vi "Sweep Control.vi"(1 "Stop":bool, 4 "Experiment Description":string="IV measurements at 0T\n- Sweep priority 0: +x gate from -10V to 10V in steps of 500mV (-x 10 to -10)\n- priority 1:+y gate from -10V to 10V in steps of 500mV (-y 10 to -10)\n- 1 IV curves at each Vsg\n- KH channel 17,18,19,20: leads 3,8,15,21\n- 5 s wait\n\nVbg = lead 26: 0V\nT: 20mK\nB=0T\n\nhash device\n\nKH channel 10,13: leads 16,27 , current mode, 5k resistor, 1000x gain\nlead 16: 3mV ac+ 1mV dc bias, 1 Hz\nKH channel 11,12: V1+/-: 17/20, 100x gain\nKH channel 5: dV: 17-20, 100x gain\n\nstripe device\n\nKH channel 7,8: leads 11,12 , current mode, 5k resistor, 1000x gain\nlead 12: 3.5mV ac+ 0mV dc bias, 1 Hz\nKH channel 6,9: V1+/-: 9,13, 100x gain\nKH channel 16: dV: 11-12, 100x gain", 5 "Experiment subVI":T6, 7 "Experiment Folder (## - Description)":string="35-2D_0T_IV_hash_stripe", 8 "error in (no error)":errorcluster, 9 "Post action (indexing priority)":T7=[enum."Do Nothing", enum."Do Nothing", enum."Do Nothing", enum."Do Nothing"], 10 "Scan parameters":T8=[{"Start"=0.0, "End"=0.0, "Step"=0.0, "Rate"=0.0, "Waveform type"=enum."linear", "wait (ms or K)"=0.0, "Address"="Dev2/ao0", "channel"=17}, {"Start"=0.0, "End"=0.0, "Step"=0.0, "Rate"=0.0, "Waveform type"=enum."linear", "wait (ms or K)"=0.0, "Address"="Dev2/ao0", "channel"=18}, {"Start"=0.0, "End"=0.0, "Step"=0.0, "Rate"=0.0, "Waveform type"=enum."linear", "wait (ms or K)"=0.0, "Address"="Dev2/ao0", "channel"=19}, {"Start"=0.0, "End"=0.0, "Step"=0.0, "Rate"=0.0, "Waveform type"=enum."linear", "wait (ms or K)"=0.0, "Address"="Dev2/ao0", "channel"=20}] {"Rate" format="%.2f"; "Step" format="%#_6p"; "End" format="%#_6p"; "Start" format="%#_6p"}, 11 "Scan control":T10=[{"Priority"=enum."Priority 0", "Scan name"=enum."Lockin Bias"}, {"Priority"=enum."Priority 1", "Scan name"=enum."Lockin Bias"}, {"Priority"=enum."Priority 0", "Scan name"=enum."Lockin Bias"}, {"Priority"=enum."Priority 1", "Scan name"=enum."Lockin Bias"}]) -> (0 "error out":errorcluster)   [LabVIEW 2019, in "Sweep Control.lvclass"]
doc: "- Priority 0 is the fastest loop\n- You can put multiple scan names in one priority.\n- OFF has to be the last priority\n- Choose an Experiment (Lockin_Sweep, IV, etc) to run at each Scan Setting\n- Open the Exeriment subVIs to choose settings"
uses:
  Sweep Control.lvclass
  Typedefs/Enum - Priority.ctl
  Typedefs/Enum - Action.ctl
  Typedefs/Cluster - ScanControl.ctl
  Typedefs/ScanControl.ctl
  Typedefs/Cluster - ScanParamters.ctl
  Typedefs/ScanParamters.ctl
  Typedefs/Enum - Experiments.ctl
  Typedefs/Sweep Control JSON--Cluster.ctl
  <userlib>/LevyLab/Transport/Control Experiment/Control Experiment.lvclass
  <userlib>/LevyLab/Transport/Transport/Transport.lvclass
  61c560dc-d997-4a5c-883d-5fdd7af828d2.vi
  Typedefs/PostAction.ctl
  Typedefs/Enum - PostAction.ctl
  Typedefs/Cluster - Sweep Control.ctl
  <userlib>/LevyLab/Transport/Transport/Typedefs/Lockin_Sweep JSON--Cluster.ctl
panel:
  in  "Lockin_Sweep Configuration":T1[](array[typedef]) {"sweepTables"."Table" format="%#_3p"; "sweepTables"."Ch" min=1 max=16; "sweepChannels"."Table" format="%#_1f"; "sweepChannels"."Channel" min=1 max=128; "sweepChannels"."Start" format="%#_6p"; "sweepChannels"."End" format="%#_6p"}
  out "Repeat #":i32
  in  "Repeat Experiment":i32=1 caption="Repeat Experiment (at each parameter)" min=1
  in  "Scan parameters 2":T2[](array[typedef]) {"Rate" format="%.2f"; "Step" format="%#_6p"; "End" format="%#_6p"; "Start" format="%#_6p"}
  # "1. Scan Parameters. Choose parameters at which each experiment will take place."
  # "2. Experiment"
  # "3. If your chosen experiment is \"Lockin Sweep\", then the following sequence of sweeps will be executed at each scan parameter. (Ex. 1. Set B. 2. Set Set Vsg. 3. Lockin Sweep 1. 4. Lockin Sweep 2. Etc."
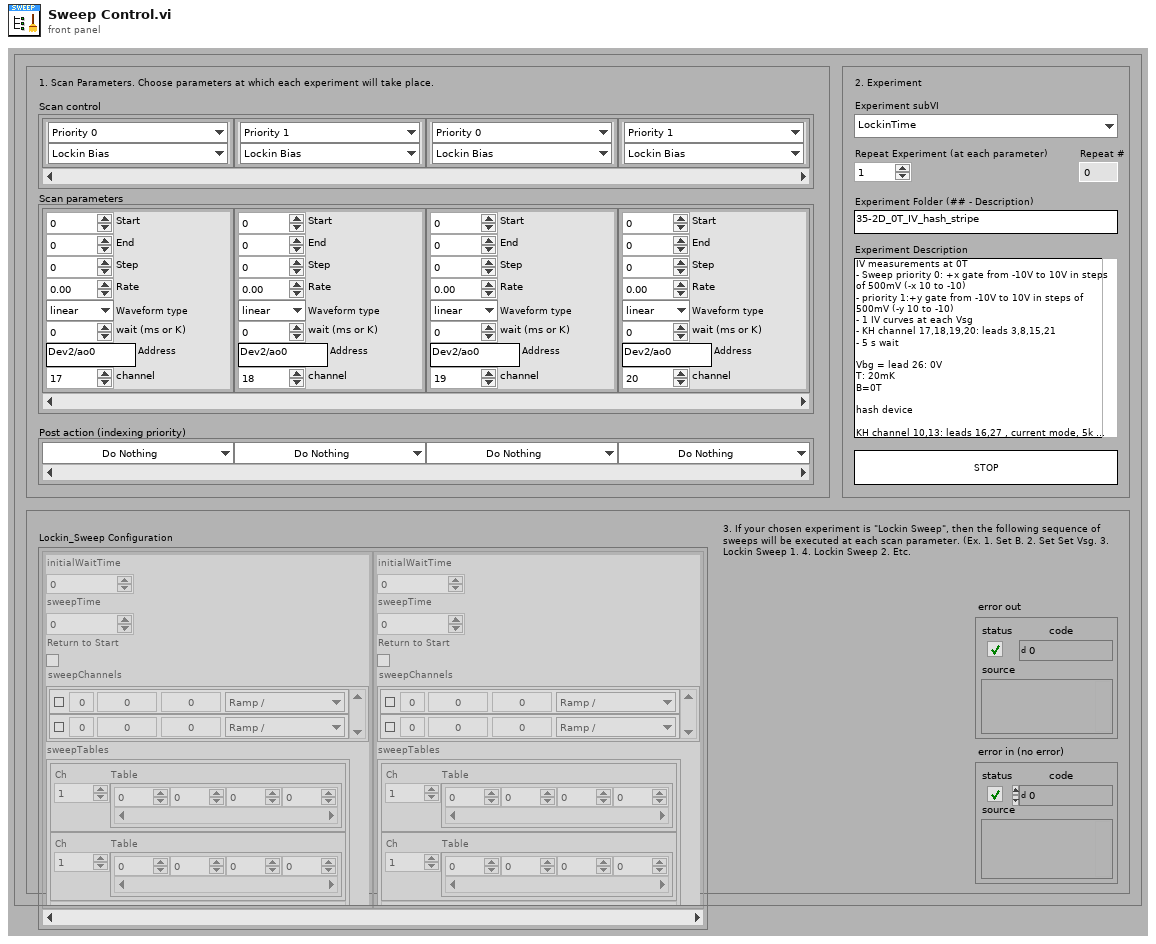
[diagram p1: front panel]
types:
  T1 = typedef "Transport.lvclass/Lockin_Sweep JSON--Cluster.ctl" = cluster{"initialWaitTime":dbl, "sweepTime":dbl, "Return to Start":bool, "sweepChannels":cluster{"Enable?":bool, "Channel":u16, "Start":dbl, "End":dbl, "Pattern":enum16{"Ramp /", "Ramp /\\", "Smooth Ramp _/", "Smooth Ramp _/\\_", "Table"}, "Table":dbl[]}[], "sweepTables":cluster{"Ch":i32, "Table":dbl[]}[]}
  T2 = typedef "Sweep Control.lvclass/Cluster - Sweep Control.ctl" = cluster{"Start":dbl, "End":dbl, "Step":dbl, "Rate":dbl, "wait (ms/mK)":u32, "Address":string, "Priority":T3, "Scan name":T4, "Post Actions":T5[], "channel":i32}
  T3 = typedef "Sweep Control.lvclass/Enum - Priority.ctl" = enum16{"Priority 0", "Priority 1", "Priority 2", "Priority 3", "Priority 4", "Priority 5"}
  T4 = typedef "Sweep Control.lvclass/Enum - Action.ctl" = enum16{"OFF", "time", "Lockin Amplitude", "Lockin Frequency", "Lockin Bias", "Delay", "Strain", "DAQ Bias", "Magnet Field", "Temperature", "MW f1", "MW f2", "MW Amplitude1", "MW Amplitude2"}
  T5 = typedef "Sweep Control.lvclass/Enum - PostAction.ctl" = enum16{"Do Nothing", "Wait (time)", "Wait (Temperature)", "Wait (<T ; B sweep)", "Wait (Magnet)"}
  T6 = typedef "Sweep Control.lvclass/Enum - Experiments.ctl" = enum16{"LockinTime", "LockinSweep", "LockinDelayLine"}
  T7 = typedef "Sweep Control.lvclass/PostAction.ctl" = T5[]
  T8 = typedef "Sweep Control.lvclass/ScanParamters.ctl" = T9[]
  T9 = typedef "Sweep Control.lvclass/Cluster - ScanParamters.ctl" = cluster{"Start":dbl, "End":dbl, "Step":dbl, "Rate":dbl, "Waveform type":enum16{"linear", "triangle", "power"}, "wait (ms or K)":dbl, "Address":string, "channel":i32}
  T10 = typedef "Sweep Control.lvclass/ScanControl.ctl" = T11[]
  T11 = typedef "Sweep Control.lvclass/Cluster - ScanControl.ctl" = cluster{"Priority":T3, "Scan name":T4}
  T12 = enum32{"Invalid", "Standard", "Closed", "Hidden", "Minimized", "Maximized"}
  T13 = enum32{"invalid app kind", "Development System", "Run Time System", "Student Edition", "Embedded LabVIEW", "Evaluation", "Custom"}
  T14 = typedef "Sweep Control.lvclass/Sweep Control JSON--Cluster.ctl" = cluster{"Experiment":T6, "Repeat Experiment":i32, "Scan control":T10, "Scan parameters":T8}
  T15 = cluster{"Core":cluster{"Current VI Reference":refnum<vi>, "Close Panel on Exit?":bool}, "SweepControl":refnum<class "Sweep Control.lvclass">, "SweepControl_JSON":T14}
  T16 = cluster{"Current VI Reference":refnum<vi>, "Close Panel on Exit?":bool}
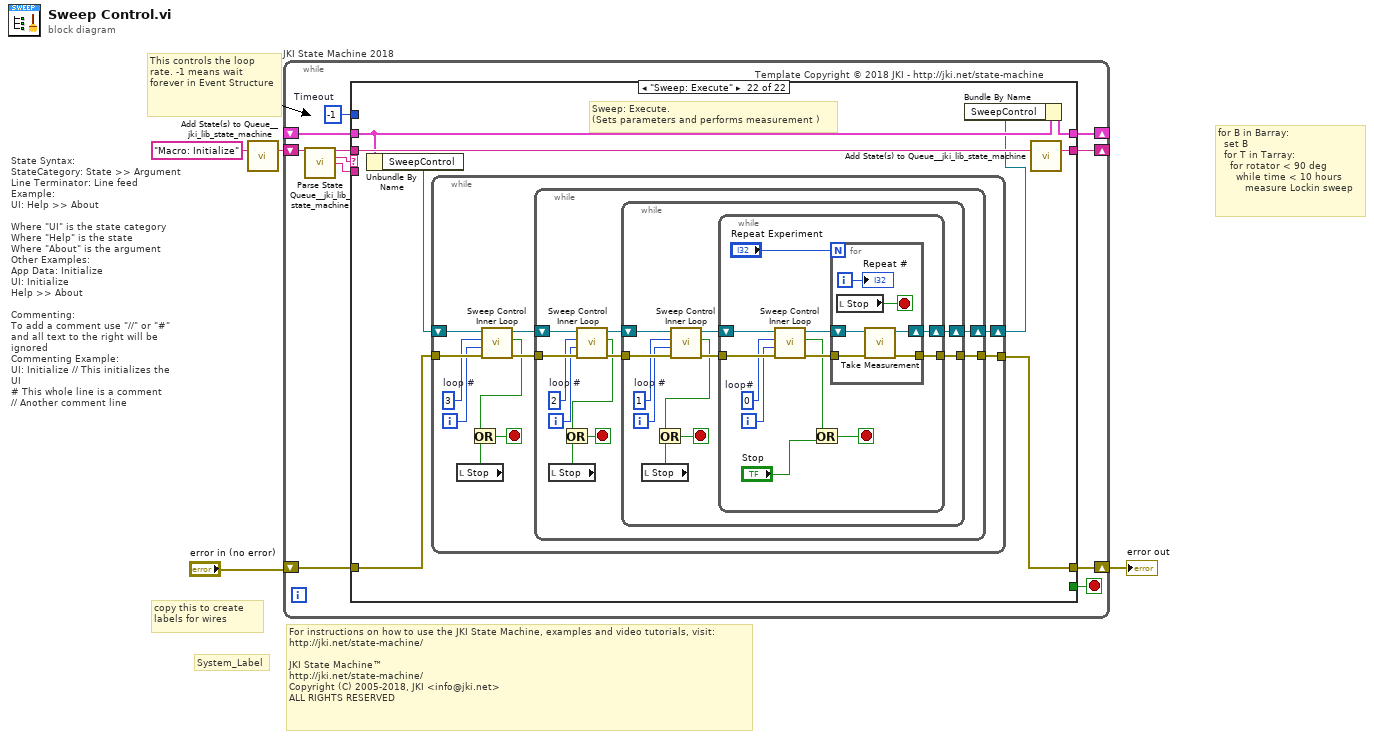
[diagram p0: block diagram]
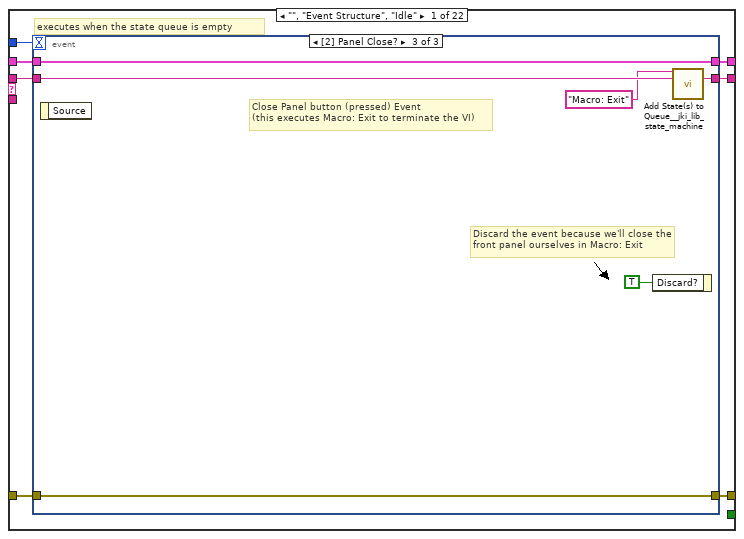
[diagram p2: hidden frame]
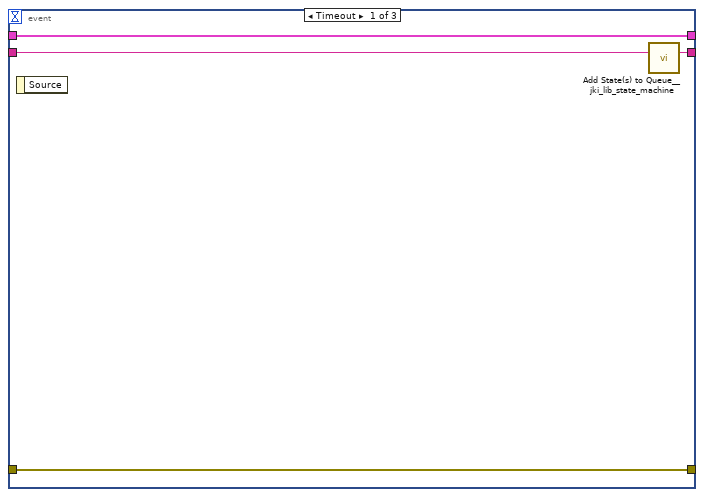
[diagram p3: hidden frame]
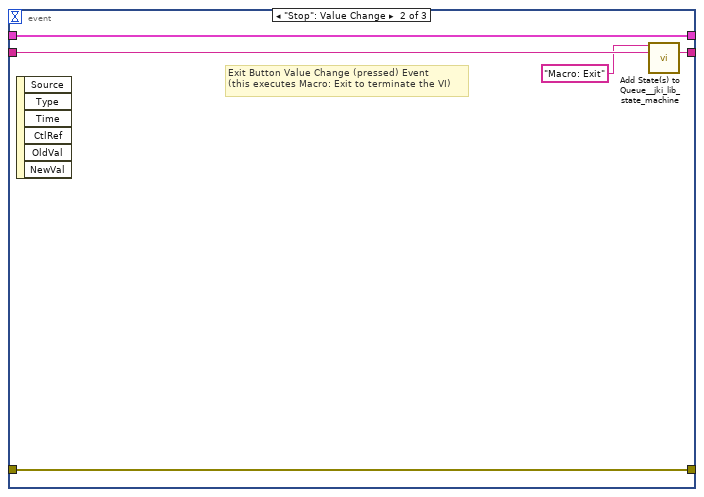
[diagram p4: hidden frame]
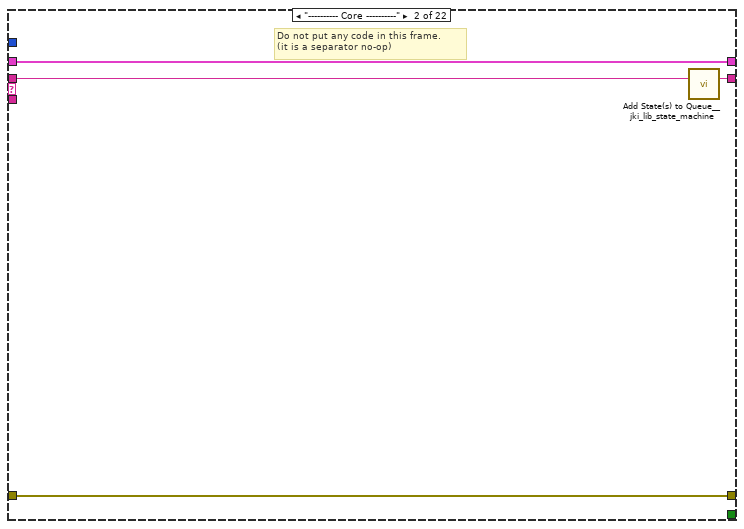
[diagram p5: hidden frame]
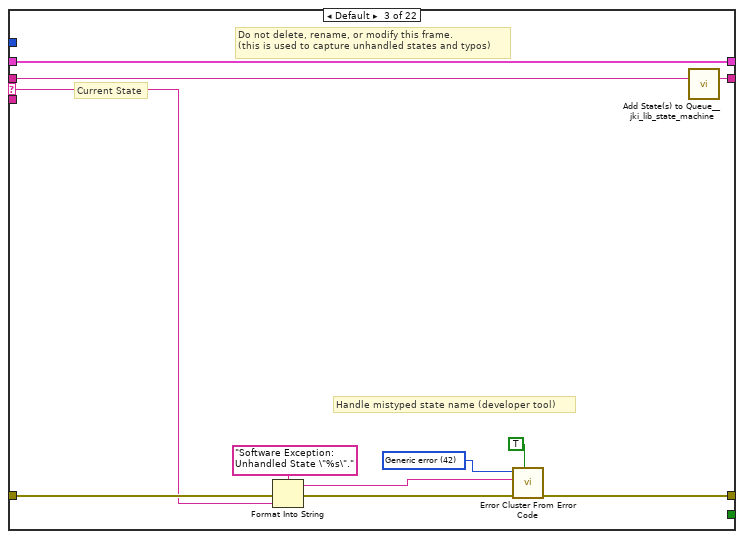
[diagram p6: hidden frame]
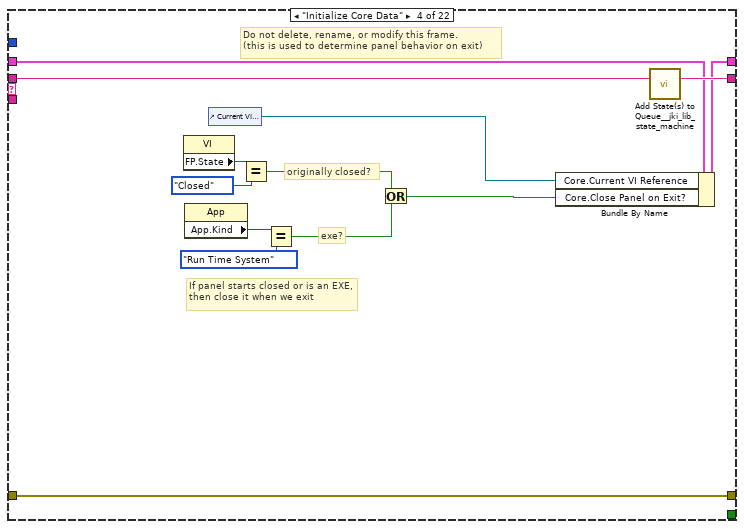
[diagram p7: hidden frame]
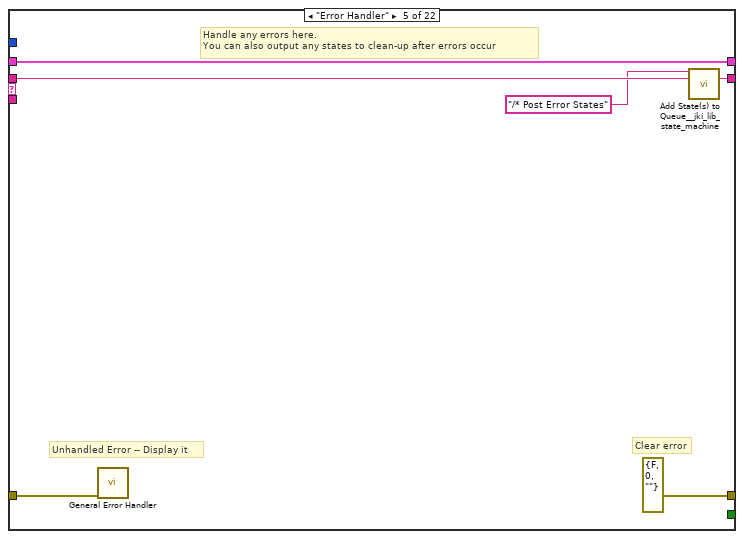
[diagram p8: hidden frame]
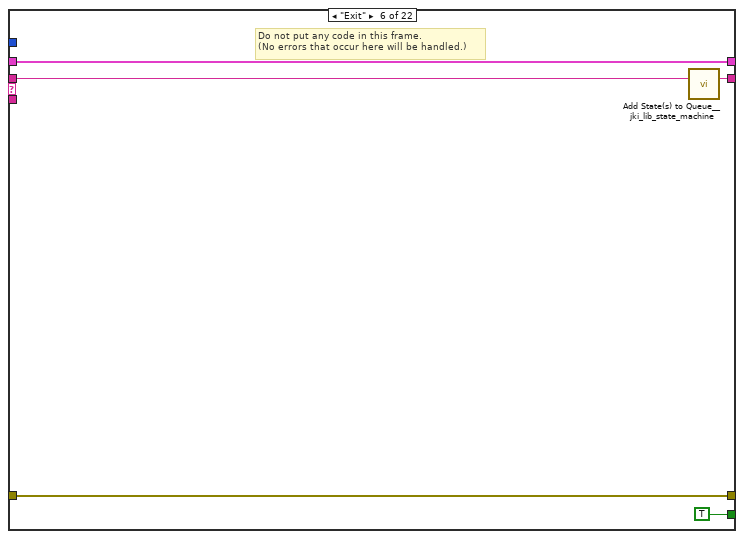
[diagram p9: hidden frame]
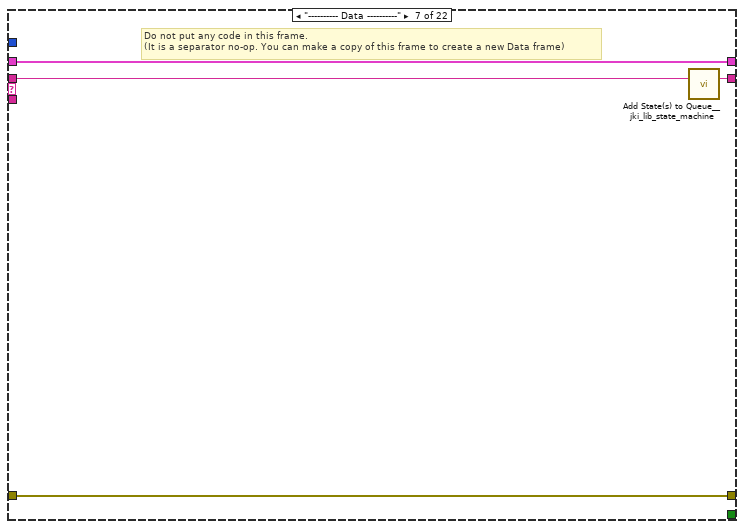
[diagram p10: hidden frame]
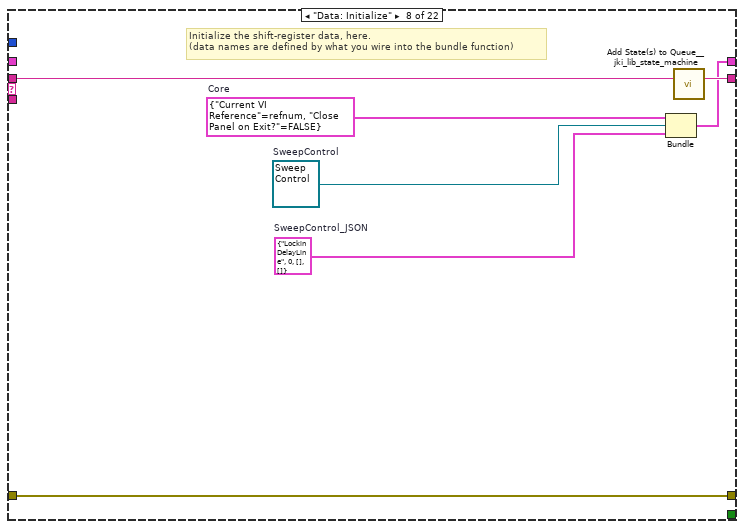
[diagram p11: hidden frame]
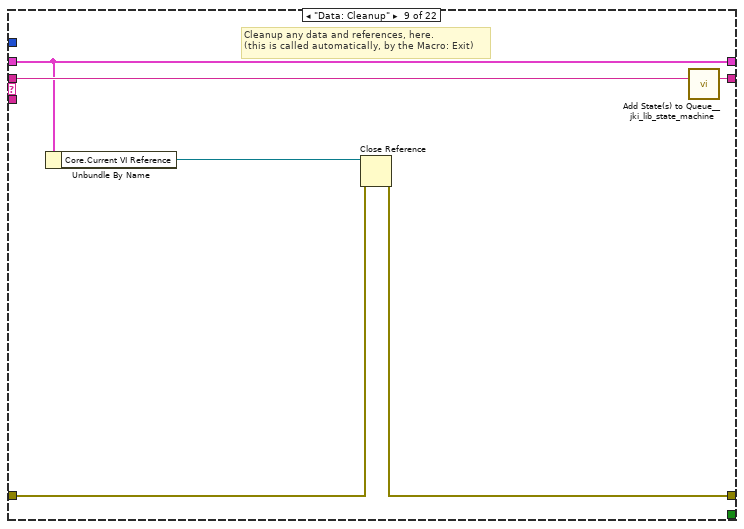
[diagram p12: hidden frame]
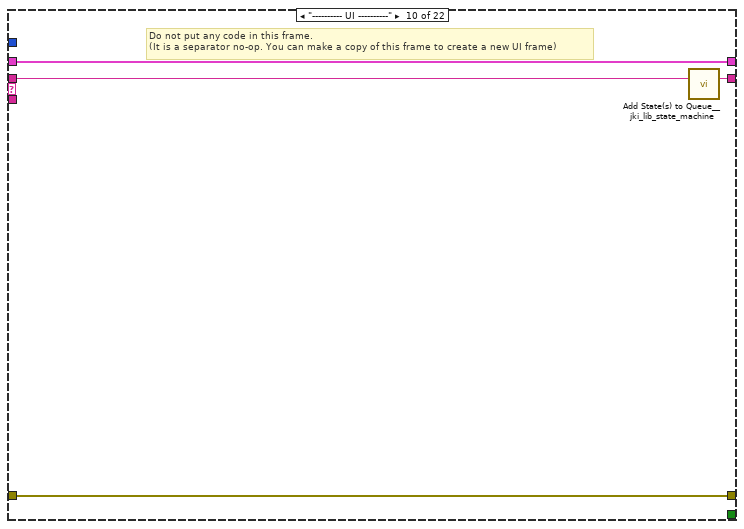
[diagram p13: hidden frame]
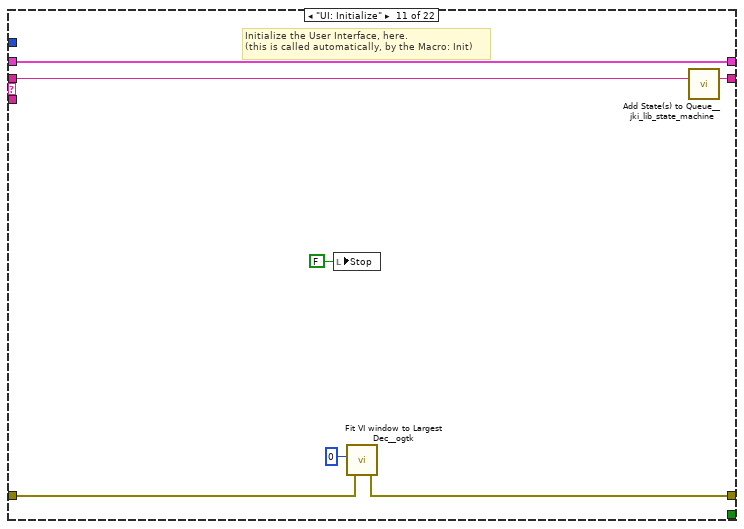
[diagram p14: hidden frame]
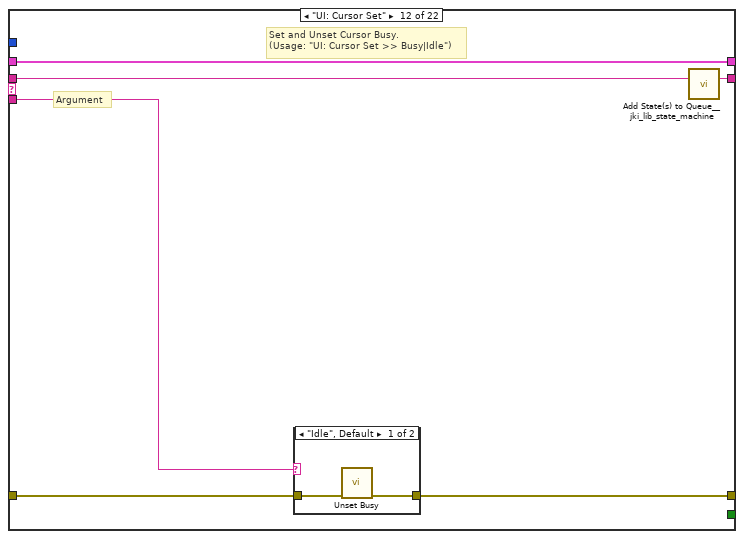
[diagram p15: hidden frame]
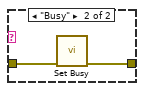
[diagram p16: hidden frame]
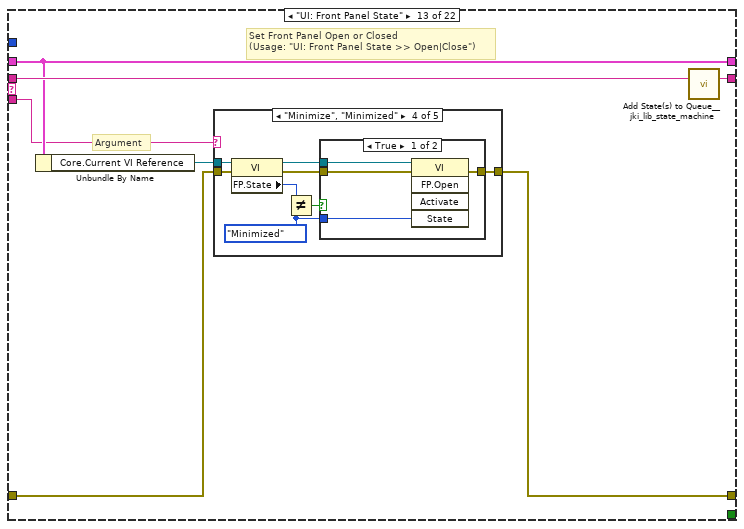
[diagram p17: hidden frame]
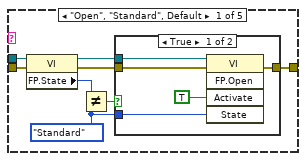
[diagram p18: hidden frame]
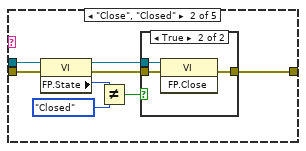
[diagram p20: hidden frame]
diagram:
  # "for B in Barray:\n  set B\n  for T in Tarray:\n    for rotator < 90 deg\n      while time < 10 hours\n         measure Lockin sweep"
  # "For instructions on how to use the JKI State Machine, examples and video tutorials, visit:\nhttp://jki.net/state-machine/\n\nJKI State Machine™\nhttp://jki.net/state-machine/\nCopyright (C) 2005-2018, JKI <info@jki.net>\nALL RIGHTS RESERVED"
  # "State Syntax:\nStateCategory: State >> Argument\nLine Terminator: Line feed\nExample:\nUI: Help >> About\n\nWhere \"UI\" is the state category\nWhere \"Help\" is the state\nWhere \"About\" is the argument\nOther Examples:\nApp Data: Initialize\nUI: Initialize\nHelp >> About\n\nCommenting:\nTo add a comment use \"//\" or \"#\" and all text to the right will be ignored\nCommenting Example:\nUI: Initialize // This initializes the UI\n# This whole line is a comment\n// Another comment line"
  # "copy this to create labels for wires"
  # "This controls the loop rate. -1 means wait forever in Event Structure"
  # "System_Label"
  n1 = call <vilib>:"Add State(s) to Queue__jki_lib_state_machine.vi"("State(s) in (\"\")"="Macro: Initialize") -> ("States Out"=w4:string)  [unwired: 14 in]
  n2 = while "JKI State Machine 2018" {
    shift-right: [w8] -> _
    shift-left: _ -> [w7]
    shift-right: [w11] -> w1
    shift-left: "error in (no error)" -> [w5]
    shift-right: [w10] -> _
    shift-left: w4 -> [w12]
    stop <- w9 stop-if-true
    w6 = -1  # Timeout
    # "Template Copyright © 2018 JKI - http://jki.net/state-machine"
    n3 = call <vilib>:"Parse State Queue__jki_lib_state_machine.vi"("State Queue"=w12) -> ("Remaining States"=w14:string, "Current State"=w15:string, "Arguments"=w13:string)  [unwired: 12 in]
    n4 = case shown="\"Sweep: Execute\"" w15 {
      selector: w15 -> [_ _ w42 _ _ _ _ _ _ _ _ _ _ _ _ _ _ _ _ _ _ _]
      tunnel: w14 -> [w22 w41 w46 w65 w71 w76 w80 w87 w93 w97 w104 w110 w121 w190 w195 w200 w211 w215 w244 w254 w278 w285]
      tunnel: w13 -> [_ _ _ _ _ _ _ _ _ _ _ w105 w115 _ _ _ _ _ _ _ _ _]
      tunnel: w7 -> [w20 w38 w44 w58 w68 w74 w77 _ w88 w94 w102 w108 w117 w187 w192 w197 w208 w212 w241 w250 w263 w283]
      tunnel: [w19 w39 w48 w62 errorcluster {"status"=FALSE, "code"=0, "source"=""} ("error out") w73 w78 w84 w89 w95 w99 w106 w118 w188 w193 w198 w209 w213 w239 w252 w265 w280] -> w11
      tunnel: w5 -> [w18 w39 w47 w62 w67 w73 w78 w84 w90 w95 w98 w107 w119 w188 w193 w198 w209 w213 w237 w252 w257 w279]
      tunnel: [w21 w40 w45 w64 w70 w75 w79 w86 w92 w96 w103 w109 w120 w189 w194 w199 w210 w214 w243 w253 w277 w286] -> w10
      tunnel: [_ _ _ _ _ TRUE _ _ _ _ _ _ _ _ _ _ _ _ _ _ _ _] -> w9
      tunnel: [w17 w38 w44 w63 w68 w74 w77 w85 w88 w94 w102 w108 w117 w187 w192 w197 w208 w212 w240 w251 w264 w282] -> w8
      tunnel: w6 -> [w16 _ _ _ _ _ _ _ _ _ _ _ _ _ _ _ _ _ _ _ _ _]
      frame "", "Event Structure", "Idle" {
        # "executes when the state queue is empty"
        n5 = event shown="[2] Panel Close?" {
          selector: _ -> [_ _ _]
          dyn-events: _ -> [_ _ _]
          timeout: w16 -> [_ _ _]
          tunnel: w22 -> [w26 w31 w37]
          tunnel: [w25 w30 w36] -> w21
          tunnel: w20 -> [w23 w28 w34]
          tunnel: [w24 w29 w35] -> w19
          tunnel: w18 -> [w24 w29 w35]
          tunnel: [w23 w28 w34] -> w17
          event Timeout {
            n6 = event-data() -> ()  [unwired: 1 in, 1 out]
            n7 = call <vilib>:"Add State(s) to Queue__jki_lib_state_machine.vi"("State(s) in (\"\")"=w26) -> ("States Out"=w25:string)  [unwired: 14 in]
          }
          event "Stop": Value Change {
            # "Exit Button Value Change (pressed) Event\n(this executes Macro: Exit to terminate the VI)"
            n8 = event-data() -> ()  [unwired: 1 in, 6 out]
            n9 = call <vilib>:"Add State(s) to Queue__jki_lib_state_machine.vi"("State(s) in Front (\"\")"="Macro: Exit", "State(s) in (\"\")"=w31) -> ("States Out"=w30:string)  [unwired: 13 in]
          }
          event Panel Close? {
            # "Discard the event because we'll close the front panel ourselves in Macro: Exit"
            # "Close Panel button (pressed) Event\n(this executes Macro: Exit to terminate the VI)"
            n10 = event-data() -> ()  [unwired: 1 in, 1 out]
            n11 = event-data("Discard?"=TRUE) -> ()  [unwired: 1 in, 1 out]
            n12 = call <vilib>:"Add State(s) to Queue__jki_lib_state_machine.vi"("State(s) in Front (\"\")"="Macro: Exit", "State(s) in (\"\")"=w37) -> ("States Out"=w36:string)  [unwired: 13 in]
          }
        }
      }
      frame "---------- Core ----------" {
        # "Do not put any code in this frame.\n(it is a separator no-op)"
        n13 = call <vilib>:"Add State(s) to Queue__jki_lib_state_machine.vi"("State(s) in (\"\")"=w41) -> ("States Out"=w40:string)  [unwired: 14 in]
      }
      frame Default {
        w51 = 42 items=["No error", "Argument error", "Memory is full", "Out of zone", "End of file", "File already open", "Generic file I/O error", "File not found", "File permission error", "Disk is full", "Duplicate path", "Too many files open", "System feature not enabled", "Resource file not found", "Cannot add resource", "Resource not found", "Image not found", "Image memory error", "Pen does not exist", "Config type invalid", "Config token not found", "Config parse error", "Config memory error", "Bad external code format", "Bad external code offset", "External code not present", "Null window", "Destroy window error", "Null menu", "Print aborted", "Bad print record", "Print driver error", "Windows error during printing", "Memory error during printing", "Print dialog error", "Generic print error", "Invalid device refnum", "Device not found", "Device parameter error", "Device unit error", "Cannot open device", "Device call aborted", "Generic error", "Cancelled by user", "Object ID too low", "Object ID too high", "Object not in heap", "Unknown heap", "Unknown object (invalid DefProc)", "Unknown object (DefProc not in table)", "Message out of range", "Invalid (null) method", "Unknown message", "Manager call not supported", "Bad address", "Network operation in progress", "Network operation timed out", "Connection is busy", "Network attribute not supported", "Network error", "Address in use", "System out of memory", "Connection aborted", "Connection refused", "Not connected", "Already connected", "Connection closed", "Initialization error (interapplication manager)", "Bad occurrence", "Wait on unbound occurrence handler", "Occurrence queue overflow", "Datalog type conflict", "Unused", "Unrecognized type (interapplication manager)", "Memory corrupt", "Failed to make temporary DLL", "Old CIN version", "Drag socket not found", "Failed to load drop-object", "Failed to register OLE object", "Failed to release OLE object", "Format specifier type mismatch", "Unknown format specifier", "Too few format specifiers", "Too many format specifiers", "Scan failed", "Newer CIN version", "Error converting to variant", "Runtime menu error", "Password tampered", "Variant attribute not found", "Incompatible variant data type", "Event data is not available", "Event Store is not present", "Occurrence is not found", "Event Queue is not created", "Event info is not available", "Refnum passed is NULL", "Error retrieving Class GUID", "Error retrieving CoClass GUID", "Error retrieving TypeLib GUID.", "Bad built application magic bytes.", "Specific driver is different from the specific driver associated with the Logical Name.", "There is no session opened to the class driver.", "Max Error", "MAX - Error with config objects", "MAX - Error loading configuration", "MAX - Group not supported"]
        # "Current State"
        # "Do not delete, rename, or modify this frame.\n(this is used to capture unhandled states and typos)"
        # "Handle mistyped state name (developer tool)"
        n14 = Format Into String(format string="Software Exception: Unhandled State \"%s\"." ("message"), error in=w47, w42) -> (resulting string=w50:string, error out=w49:errorcluster)  [unwired: 1 in]
        n15 = call <vilib>:"Error Cluster From Error Code.vi"("show call chain? (False)"=TRUE, "error in (no error)"=w49, "error message (\"\")"=w50, "error code (0)"=w51) -> ("error out"=w48:errorcluster)  [unwired: 5 in]
        n16 = call <vilib>:"Add State(s) to Queue__jki_lib_state_machine.vi"("State(s) in (\"\")"=w46) -> ("States Out"=w45:string)  [unwired: 14 in]
      }
      frame "Initialize Core Data" {
        # "Do not delete, rename, or modify this frame.\n(this is used to determine panel behavior on exit)"
        # "originally closed?"
        # "exe?"
        # "If panel starts closed or is an EXE, then close it when we exit"
        n17 = property class="VI"() -> ("FP.State"=w55:T12)  [unwired: 2 in, 2 out]
        n18 = property class="App"() -> ("App.Kind"=w61:T13)  [unwired: 2 in, 2 out]
        n19 = control-ref of="Current VI Reference"() -> (w56:refnum<vi>)
        n20 = Equal?(x=w55, y=T12."Closed" ("Front Panel Window:State")) -> (x = y?=w53:bool)
        n21 = Equal?(x=w61, y=T13."Run Time System" ("Application:Kind")) -> (x = y?=w59:bool)
        n22 = Or(x=w53, y=w59) -> (x .or. y?=w57:bool)
        n23 = Bundle By Name(cluster=w58, "Core.Current VI Reference"=w56, "Core.Close Panel on Exit?"=w57) -> (w63:T15)
        n24 = call <vilib>:"Add State(s) to Queue__jki_lib_state_machine.vi"("State(s) in (\"\")"=w65) -> ("States Out"=w64:string)  [unwired: 14 in]
      }
      frame "Error Handler" {
        # "Unhandled Error -- Display it"
        # "Handle any errors here.\nYou can also output any states to clean-up after errors occur"
        # "Clear error"
        n25 = call <vilib>:"General Error Handler.vi"("error in (no error)"=w67) -> ()  [unwired: 10 in, 5 out]
        n26 = call <vilib>:"Add State(s) to Queue__jki_lib_state_machine.vi"("State(s) in Front (\"\")"="/* Post Error States", "State(s) in (\"\")"=w71) -> ("States Out"=w70:string)  [unwired: 13 in]
      }
      frame "Exit" {
        # "Do not put any code in this frame.\n(No errors that occur here will be handled.)"
        n27 = call <vilib>:"Add State(s) to Queue__jki_lib_state_machine.vi"("State(s) in (\"\")"=w76) -> ("States Out"=w75:string)  [unwired: 14 in]
      }
      frame "---------- Data ----------" {
        # "Do not put any code in this frame.\n(It is a separator no-op. You can make a copy of this frame to create a new Data frame)"
        n28 = call <vilib>:"Add State(s) to Queue__jki_lib_state_machine.vi"("State(s) in (\"\")"=w80) -> ("States Out"=w79:string)  [unwired: 14 in]
      }
      frame "Data: Initialize" {
        w81 = T14 {"Experiment"=enum."LockinDelayLine", "Repeat Experiment"=0, "Scan control"=[], "Scan parameters"=[]}  # SweepControl_JSON
        w82 = refnum<class "Sweep Control.lvclass"> refnum  # SweepControl
        w83 = T16 {"Current VI Reference"=refnum, "Close Panel on Exit?"=FALSE}  # Core
        # "Initialize the shift-register data, here.\n(data names are defined by what you wire into the bundle function)"
        n29 = Bundle("Core"=w83, "SweepControl"=w82, "SweepControl_JSON"=w81) -> (w85:T15)  [unwired: 1 in]
        n30 = call <vilib>:"Add State(s) to Queue__jki_lib_state_machine.vi"("State(s) in (\"\")"=w87) -> ("States Out"=w86:string)  [unwired: 14 in]
      }
      frame "Data: Cleanup" {
        # "Cleanup any data and references, here.\n(this is called automatically, by the Macro: Exit)"
        n31 = Unbundle By Name(w88) -> ("Core.Current VI Reference"=w91:refnum<vi>)
        n32 = Close Reference(reference=w91, error in (no error)=w90) -> (error out=w89:errorcluster)
        n33 = call <vilib>:"Add State(s) to Queue__jki_lib_state_machine.vi"("State(s) in (\"\")"=w93) -> ("States Out"=w92:string)  [unwired: 14 in]
      }
      frame "---------- UI ----------" {
        # "Do not put any code in this frame.\n(It is a separator no-op. You can make a copy of this frame to create a new UI frame)"
        n34 = call <vilib>:"Add State(s) to Queue__jki_lib_state_machine.vi"("State(s) in (\"\")"=w97) -> ("States Out"=w96:string)  [unwired: 14 in]
      }
      frame "UI: Initialize" {
        # "Initialize the User Interface, here.\n(this is called automatically, by the Macro: Init)"
        n35 = local write "Stop"(FALSE ("Stop")) -> ()
        n36 = call <userlib>:"Fit VI window to Largest Dec__ogtk.vi"("error in (no error)"=w98, "border spacing (2 px)"=0) -> ("error out"=w99:errorcluster)  [unwired: 4 in, 1 out]
        n37 = call <vilib>:"Add State(s) to Queue__jki_lib_state_machine.vi"("State(s) in (\"\")"=w104) -> ("States Out"=w103:string)  [unwired: 14 in]
      }
      frame "UI: Cursor Set" {
        # "Argument"
        # "Set and Unset Cursor Busy.\n(Usage: \"UI: Cursor Set >> Busy|Idle\")"
        n38 = case shown="\"Idle\", Default" w105 {
          tunnel: w107 -> [w112 w114]
          tunnel: [w111 w113] -> w106
          frame "Idle", Default {
            n39 = call <vilib>:"Unset Busy.vi"("error in (no error)"=w112) -> ("error out"=w111:errorcluster)  [unwired: 10 in]
          }
          frame "Busy" {
            n40 = call <vilib>:"Set Busy.vi"("error in (no error)"=w114) -> ("error out"=w113:errorcluster)  [unwired: 9 in, 1 out]
          }
        }
        n41 = call <vilib>:"Add State(s) to Queue__jki_lib_state_machine.vi"("State(s) in (\"\")"=w110) -> ("States Out"=w109:string)  [unwired: 14 in]
      }
      frame "UI: Front Panel State" {
        # "Argument"
        # "Set Front Panel Open or Closed\n(Usage: \"UI: Front Panel State >> Open|Close\")"
        n42 = Unbundle By Name(w117) -> ("Core.Current VI Reference"=w116:refnum<vi>)
        n43 = case shown="\"Minimize\", \"Minimized\"" w115 {
          tunnel: w119 -> [w127 w142 w153 w166 w179]
          tunnel: [w129 w143 w155 w168 w181] -> w118
          tunnel: w116 -> [w128 w140 w154 w167 w180]
          frame "Open", "Standard", Default {
            w122 = T12."Standard" ("State")
            n44 = property class="VI"(reference=w128, error in=w127) -> (reference out=w125:refnum<vi>, error out=w126:errorcluster, "FP.State"=w124:T12)
            n45 = Not Equal?(x=w124, y=w122) -> (x != y?=w123:bool)
            n46 = case shown="True" w123 {
              tunnel: [w133 w135] -> w129
              tunnel: w126 -> [w132 w135]
              tunnel: w125 -> [w131 _]
              tunnel: w122 -> [w130 _]
              frame True {
                n47 = invoke class="VI" method="FP.Open"(reference=w131, error in=w132, "Activate"=TRUE, "State"=w130) -> (error out=w133:errorcluster)  [unwired: 1 in, 4 out]
              }
              frame False {
              }
            }
          }
          frame "Close", "Closed" {
            n48 = property class="VI"(reference=w140, error in=w142) -> (reference out=w139:refnum<vi>, error out=w141:errorcluster, "FP.State"=w137:T12)
            n49 = Not Equal?(x=w137, y=T12."Closed" ("Front Panel Window:State")) -> (x != y?=w136:bool)
            n50 = case shown="True" w136 {
              tunnel: [w144 w147] -> w143
              tunnel: w141 -> [w144 w146]
              tunnel: w139 -> [_ w145]
              frame False {
              }
              frame True {
                n51 = invoke class="VI" method="FP.Close"(reference=w145, error in=w146) -> (error out=w147:errorcluster)  [unwired: 1 in, 2 out]
              }
            }
          }
          frame "Hidden", "Hide" {
            w148 = T12."Hidden" ("State")
            n52 = property class="VI"(reference=w154, error in=w153) -> (reference out=w151:refnum<vi>, error out=w152:errorcluster, "FP.State"=w150:T12)
            n53 = Not Equal?(x=w150, y=w148) -> (x != y?=w149:bool)
            n54 = case shown="True" w149 {
              tunnel: [w159 w160] -> w155
              tunnel: w152 -> [w158 w160]
              tunnel: w151 -> [w157 _]
              tunnel: w148 -> [w156 _]
              frame True {
                n55 = invoke class="VI" method="FP.Open"(reference=w157, error in=w158, "State"=w156) -> (error out=w159:errorcluster)  [unwired: 2 in, 4 out]
              }
              frame False {
              }
            }
          }
          frame "Minimize", "Minimized" {
            w161 = T12."Minimized" ("State")
            n56 = property class="VI"(reference=w167, error in=w166) -> (reference out=w164:refnum<vi>, error out=w165:errorcluster, "FP.State"=w163:T12)
            n57 = Not Equal?(x=w163, y=w161) -> (x != y?=w162:bool)
            n58 = case shown="True" w162 {
              tunnel: [w172 w173] -> w168
              tunnel: w165 -> [w171 w173]
              tunnel: w164 -> [w170 _]
              tunnel: w161 -> [w169 _]
              frame True {
                n59 = invoke class="VI" method="FP.Open"(reference=w170, error in=w171, "State"=w169) -> (error out=w172:errorcluster)  [unwired: 2 in, 4 out]
              }
              frame False {
              }
            }
          }
          frame "Maximize", "Maximized" {
            w174 = T12."Maximized" ("State")
            n60 = property class="VI"(reference=w180, error in=w179) -> (reference out=w177:refnum<vi>, error out=w178:errorcluster, "FP.State"=w176:T12)
            n61 = Not Equal?(x=w176, y=w174) -> (x != y?=w175:bool)
            n62 = case shown="True" w175 {
              tunnel: [w185 w186] -> w181
              tunnel: w178 -> [w184 w186]
              tunnel: w177 -> [w183 _]
              tunnel: w174 -> [w182 _]
              frame True {
                n63 = invoke class="VI" method="FP.Open"(reference=w183, error in=w184, "State"=w182) -> (error out=w185:errorcluster)  [unwired: 2 in, 4 out]
              }
              frame False {
              }
            }
          }
        }
        n64 = call <vilib>:"Add State(s) to Queue__jki_lib_state_machine.vi"("State(s) in (\"\")"=w121) -> ("States Out"=w120:string)  [unwired: 14 in]
      }
      frame "---------- Macro ----------" {
        # "Do not put any code in this frame.\n(It is a separator no-op. You can make a copy of this frame to create a new Macro frame)"
        n65 = call <vilib>:"Add State(s) to Queue__jki_lib_state_machine.vi"("State(s) in (\"\")"=w190) -> ("States Out"=w189:string)  [unwired: 14 in]
      }
      frame "Macro: Initialize" {
        w191 = "Data: Initialize\nInitialize Core Data\nUI: Initialize\nUI: Front Panel State >> Open\nMacro: Sweep"  # Data: Initialize Initialize Core Data UI: Initialize UI: Front Panel State >> Open Macro: Sweep
        # "Initialization Macro\n(This is called once, when the VI starts)"
        n66 = call <vilib>:"Add State(s) to Queue__jki_lib_state_machine.vi"("State(s) in Front (\"\")"=w191, "State(s) in (\"\")"=w195) -> ("States Out"=w194:string)  [unwired: 13 in]
      }
      frame "Macro: Sweep" {
        # "Macro: Sweep.\n(Initialize Sweep, Execute Sweep, Exit)"
        n67 = call <vilib>:"Add State(s) to Queue__jki_lib_state_machine.vi"("State(s) in Front (\"\")"="Sweep: Initialize\nSweep: Prepare JSON\nSweep: Write JSON\nSweep: Execute\nMacro: Exit", "State(s) in (\"\")"=w200) -> ("States Out"=w199:string)  [unwired: 13 in]
      }
      frame "Macro: Exit" {
        # "Exit Macro\n(This is called once, when the VI exits)"
        n68 = Unbundle By Name(w208) -> ("Core.Close Panel on Exit?"=w207:bool)
        n69 = Select(t="UI: Front Panel State >> Close", s=w207, f="") -> (s? t:f=w204:string)
        n70 = call <vilib>:"Add State(s) to Queue__jki_lib_state_machine.vi"("State(s) in Front (\"\")"="", "State(s) in (\"\")"=w204, "State(s) at Back (\"\")"="Data: Cleanup\nExit") -> ("States Out"=w202:string)  [unwired: 12 in]
        n71 = call <vilib>:"Add State(s) to Queue__jki_lib_state_machine.vi"("State(s) in Front (\"\")"=w202, "State(s) in (\"\")"=w211) -> ("States Out"=w210:string)  [unwired: 13 in]
      }
      frame "---------- Sweep ----------" {
        # "Template Separator\n(You can make a copy of, or modify, this frame)"
        n72 = call <vilib>:"Add State(s) to Queue__jki_lib_state_machine.vi"("State(s) in (\"\")"=w215) -> ("States Out"=w214:string)  [unwired: 14 in]
      }
      frame "Sweep: Initialize" {
        # "hidden: 1/7/2020"
        # "Sweep: Initialize.\n(Read Control Experiment.json, Sets Experiment Description and Folder, Prepare Sweep (eg, sort scan priorities))"
        n73 = Unbundle By Name(w241) -> ("SweepControl"=w219:refnum<class "Sweep Control.lvclass">)
        n74 = call <userlib>:"Control Experiment FGV.vi"("Function"=enum16{"read", "write"}."read", "error in (no error)"=w237) -> ("error out"=w233:errorcluster, "Control Experiment.lvclass out"=w235:refnum<class "Control Experiment.lvclass">)  [unwired: 6 in, 2 out]
        n75 = call <userlib>:"Write Experiment Description.vi"("error in (no error)"=w233, "Experiment Description"="Experiment Description", "Control Experiment in"=w235) -> ("error out"=w232:errorcluster, "Control Experiment out"=w231:refnum<class "Control Experiment.lvclass">)  [unwired: 7 in]
        n76 = call <userlib>:"Write Experiment Folder.vi"("error in (no error)"=w232, "Experiment Folder"="Experiment Folder (## - Description)", "Control Experiment in"=w231) -> ("error out"=w227:errorcluster, "Control Experiment out"=w228:refnum<class "Control Experiment.lvclass">)  [unwired: 7 in]
        n77 = call <userlib>:"Write Dependencies.vi"("error in (no error)"=w227, "Control Experiment"=w228) -> ("error out"=w223:errorcluster, "Transport out"=w224:refnum<class "Transport.lvclass">)  [unwired: 8 in]
        n78 = call "Create Scan.vi"("Post action (indexing priority)"="Post action (indexing priority)", "Scan parameters"="Scan parameters", "Scan control"="Scan control", "SweepControl"=w219) -> ("SweepControl"=w218:refnum<class "Sweep Control.lvclass">)  [unwired: 7 in]
        n79 = Bundle By Name(cluster=w218, "Experiment"="Experiment subVI", "Scan parameters 2"="Scan parameters 2", "Lockin_Sweep Configuration"="Lockin_Sweep Configuration") -> (w226:refnum<class "Sweep Control.lvclass">)
        n80 = call <userlib>:"Write Dependencies.vi"("error in (no error)"=w223, "Transport"=w224, "SweepControl in"=w226) -> ("error out"=w222:errorcluster, "SweepControl out"=w225:refnum<class "Sweep Control.lvclass">)  [unwired: 7 in]
        n81 = call "Sort Scan Parameters.vi"("error in (no error)"=w222, "SweepControl"=w225) -> ("error out"=w239:errorcluster, "SweepControl"=w229:refnum<class "Sweep Control.lvclass">)  [unwired: 6 in, 2 out]
        n82 = Bundle By Name(cluster=w241, "SweepControl"=w229) -> (w240:T15)
        n83 = call <vilib>:"Add State(s) to Queue__jki_lib_state_machine.vi"("State(s) in (\"\")"=w244) -> ("States Out"=w243:string)  [unwired: 14 in]
      }
      frame "Sweep: Prepare JSON" {
        # "Sweep: Prepare JSON.\n(Prepare Sweep Configuration data for *.json file)"
        n84 = Unbundle By Name(w250) -> ("SweepControl"=w249:refnum<class "Sweep Control.lvclass">)
        n85 = Unbundle By Name(w249) -> ("Scan control"=w248:T10, "Scan parameters"=w247:T8, "Experiment"=w246:T6)
        n86 = local read "Repeat Experiment"() -> (w245:i32)
        n87 = Bundle By Name(cluster=w250, "SweepControl_JSON.Scan control"=w248, "SweepControl_JSON.Scan parameters"=w247, "SweepControl_JSON.Experiment"=w246, "SweepControl_JSON.Repeat Experiment"=w245) -> (w251:T15)
        n88 = call <vilib>:"Add State(s) to Queue__jki_lib_state_machine.vi"("State(s) in (\"\")"=w254) -> ("States Out"=w253:string)  [unwired: 14 in]
      }
      frame "Sweep: Write JSON" {
        # "Sweep: Write JSON.\n(Writes <SweepControl> json section)"
        n89 = Unbundle By Name(w263) -> ("SweepControl"=w262:refnum<class "Sweep Control.lvclass">, "SweepControl_JSON"=w260:T14)
        n90 = call <userlib>:"Read Dependencies.vi"("error in (no error)"=w257, "SweepControl in"=w262) -> ("error out"=w275:errorcluster, "Transport"=w276:refnum<class "Transport.lvclass">, "SweepControl out"=w269:refnum<class "Sweep Control.lvclass">)  [unwired: 7 in]
        n91 = call <userlib>:"Read Dependencies.vi"("error in (no error)"=w275, "Transport"=w276) -> ("error out"=w256:errorcluster, "C.E."=w259:refnum<class "Control Experiment.lvclass">, "Transport"=w270:refnum<class "Transport.lvclass">)  [unwired: 7 in]
        n92 = call <userlib>:"Write JSON to Dictionary.vi"("error in (no error)"=w256, "Control Experiment in"=w259) -> ("error out"=w255:errorcluster, "Control Experiment out"=w258:refnum<class "Control Experiment.lvclass">)  [unwired: 8 in]
        n93 = call "To JSON Text.vim"("error in (no error)"=w255, "Anything"=w260) -> ("error out"=w272:errorcluster, "<JSON>"=w274:string)  [unwired: 8 in]
        n94 = call <userlib>:"Write Dictionary Element.vi"("error in (no error)"=w272, "value"=w274, "key"="<SweepControl>", "Control Experiment in"=w258) -> ("error out"=w267:errorcluster, "Control Experiment out"=w271:refnum<class "Control Experiment.lvclass">)  [unwired: 6 in]
        n95 = call <userlib>:"Write Dependencies.vi"("error in (no error)"=w267, "Control Experiment"=w271, "Transport in"=w270) -> ("error out"=w266:errorcluster, "Transport out"=w268:refnum<class "Transport.lvclass">)  [unwired: 7 in]
        n96 = call <userlib>:"Write Dependencies.vi"("error in (no error)"=w266, "Transport"=w268, "SweepControl in"=w269) -> ("error out"=w265:errorcluster, "SweepControl out"=w261:refnum<class "Sweep Control.lvclass">)  [unwired: 7 in]
        n97 = Bundle By Name(cluster=w263, "SweepControl"=w261) -> (w264:T15)
        n98 = call <vilib>:"Add State(s) to Queue__jki_lib_state_machine.vi"("State(s) in (\"\")"=w278) -> ("States Out"=w277:string)  [unwired: 14 in]
      }
      frame "Sweep: Execute" {
        # "Sweep: Execute.\n(Sets parameters and performs measurement )"
        n99 = Unbundle By Name(w283) -> ("SweepControl"=w284:refnum<class "Sweep Control.lvclass">)
        n100 = while {
          tunnel: w279 -> [w295]
          shift-right: [w288] -> w281
          shift-left: w284 -> [w297]
          tunnel: [w287] -> w280
          i -> [w292]
          stop <- w289 stop-if-true
          w293 = 3  # loop #
          n101 = local read "Stop"() -> (w291:bool)
          n102 = call "Sweep Control Inner Loop.vi"("error in (no error)"=w295, "inner loop index"=w292, "loop #"=w293, "SweepControl in"=w297) -> ("error out"=w294:errorcluster, "Stop?"=w290:bool, "SweepControl out"=w296:refnum<class "Sweep Control.lvclass">)  [unwired: 5 in]
          n103 = Or(x=w290, y=w291) -> (x .or. y?=w289:bool)
          n104 = while {
            tunnel: w294 -> [w307]
            shift-right: [w299] -> w288
            shift-left: w296 -> [w308]
            tunnel: [w298] -> w287
            i -> [w303]
            stop <- w300 stop-if-true
            w306 = 2  # loop #
            n105 = local read "Stop"() -> (w302:bool)
            n106 = call "Sweep Control Inner Loop.vi"("error in (no error)"=w307, "inner loop index"=w303, "loop #"=w306, "SweepControl in"=w308) -> ("error out"=w305:errorcluster, "Stop?"=w301:bool, "SweepControl out"=w304:refnum<class "Sweep Control.lvclass">)  [unwired: 5 in]
            n107 = Or(x=w301, y=w302) -> (x .or. y?=w300:bool)
            n108 = while {
              tunnel: w305 -> [w319]
              shift-right: [w310] -> w299
              shift-left: w304 -> [w318]
              tunnel: [w309] -> w298
              i -> [w314]
              stop <- w311 stop-if-true
              w317 = 1  # loop #
              n109 = local read "Stop"() -> (w313:bool)
              n110 = call "Sweep Control Inner Loop.vi"("error in (no error)"=w319, "inner loop index"=w314, "loop #"=w317, "SweepControl in"=w318) -> ("error out"=w316:errorcluster, "Stop?"=w312:bool, "SweepControl out"=w315:refnum<class "Sweep Control.lvclass">)  [unwired: 5 in]
              n111 = Or(x=w312, y=w313) -> (x .or. y?=w311:bool)
              n112 = while {
                tunnel: w316 -> [w331]
                shift-right: [w323] -> w310
                shift-left: w315 -> [w327]
                tunnel: [w320] -> w309
                i -> [w322]
                stop <- w325 stop-if-true
                w330 = 0  # loop#
                n113 = call "Sweep Control Inner Loop.vi"("error in (no error)"=w331, "inner loop index"=w322, "loop #"=w330, "SweepControl in"=w327) -> ("error out"=w329:errorcluster, "Stop?"=w321:bool, "SweepControl out"=w328:refnum<class "Sweep Control.lvclass">)  [unwired: 5 in]
                n114 = Or(x=w321, y="Stop") -> (x .or. y?=w325:bool)
                n115 = for {
                  N: "Repeat Experiment" -> [_]
                  tunnel: w329 -> [w337]
                  shift-right: [w333] -> w323
                  shift-left: w328 -> [w336]
                  tunnel: [w332] -> w320
                  i -> [w335]
                  stop <- w334 stop-if-true
                  n116 = local read "Stop"() -> (w334:bool)
                  n117 = call "Take Measurement.vi"("error in (no error)"=w337, "SweepControl in"=w336) -> ("error out"=w332:errorcluster, "SweepControl"=w333:refnum<class "Sweep Control.lvclass">)  [unwired: 8 in]
                  "Repeat #" <- w335
                }
              }
            }
          }
        }
        n118 = Bundle By Name(cluster=w283, "SweepControl"=w281) -> (w282:T15)
        n119 = call <vilib>:"Add State(s) to Queue__jki_lib_state_machine.vi"("State(s) in (\"\")"=w285) -> ("States Out"=w286:string)  [unwired: 14 in]
      }
    }
  }
  "error out" <- w1
